vi "Restore Configuration.vi"(8 "error in (no error)":errorcluster, 10 "File path":path, 11 "Measure Object in":refnum<class "Template Module.lvclass">) -> (0 "error out":errorcluster, 1 "Section out":string, 2 "File path out":path, 3 "Measure Object out":refnum<class "Template Module.lvclass">)   [LabVIEW 2016, in "Template Module.lvclass"]
uses:
  Template Module.lvclass
  Template Module.lvclass/Template Module.ctl
  Read Name.vi
  Template Module Messages/Restore Configuration Msg/Restore Configuration Msg.lvclass
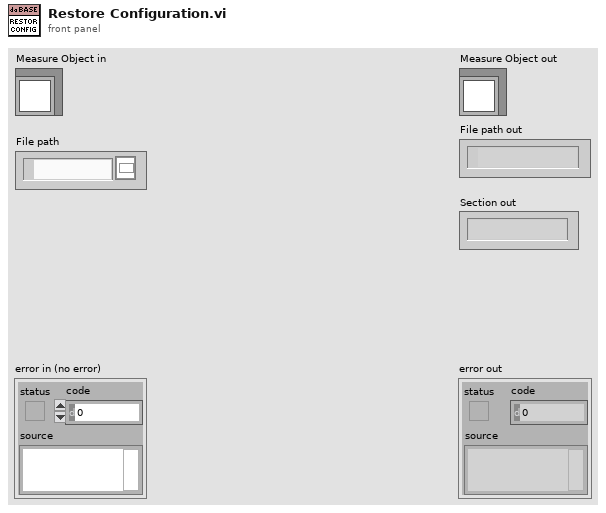
[diagram p1: front panel]
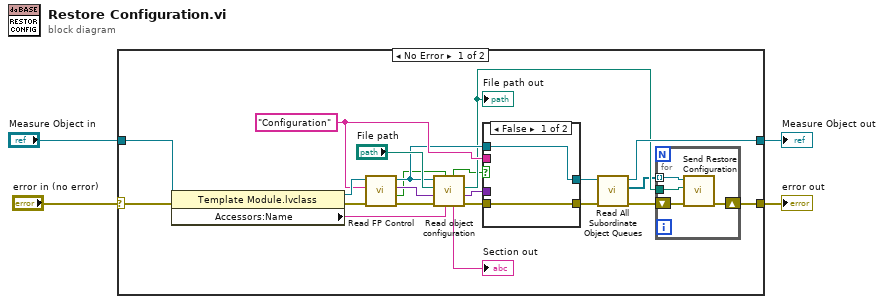
[diagram p0: block diagram]
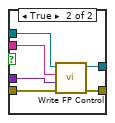
[diagram p2: hidden frame]
diagram:
  n1 = case shown="No Error" "error in (no error)" {
    selector: "error in (no error)" -> [w22 w40]
    tunnel: [w8 w40] -> w3
    tunnel: [w12 w39] -> w1
    tunnel: "Measure Object in" -> [w21 w39]
    frame No Error {
      w18 = "Configuration" ("Control Name")
      n2 = property class="Template Module.lvclass"(reference=w21, error in=w22) -> (reference out=w20:refnum<class "Template Module.lvclass">, error out=w23:errorcluster, "Accessors:Name"=w19:string)
      n3 = call-dynamic "Read FP Control.vi"("error in (no error)"=w23, "Control Name"=w18, "Measure Object in"=w20) -> ("error out"=w24:errorcluster, "Present"=w5:bool, "Control Value"=w26:variant, "Measure Object out"=w15:refnum<class "Template Module.lvclass">)  [unwired: 5 in]
      n4 = call "Read object configuration.vi"("Object name"=w19, "Present"=w5, "Error In"=w24, "type"=w26, "File path"="File path", "object"=w15) -> ("Error Out"=w16:errorcluster, "Configuration"=w17:variant, "File path out"=w11:path, "Section out"=→"Section out":string, "found?"=w6:bool)  [unwired: 1 in]
      "File path out" <- w11
      n5 = case shown="False" w6 {
        tunnel: w18 -> [_ w34]
        tunnel: w17 -> [_ w33]
        tunnel: w16 -> [w28 w32]
        tunnel: w15 -> [w27 w31]
        tunnel: [w28 w30] -> w14
        tunnel: [w27 w29] -> w13
        frame False {
        }
        frame True {
          n6 = call-dynamic "Write FP Control.vi"("error in (no error)"=w32, "Control Value"=w33, "Control Name"=w34, "Measure Object in"=w31) -> ("error out"=w30:errorcluster, "Measure Object out"=w29:refnum<class "Template Module.lvclass">)  [unwired: 6 in]
        }
      }
      n7 = call-dynamic "Read All Subordinate Object Queues.vi"("error in (no error)"=w14, "Measure Object in"=w13) -> ("error out"=w9:errorcluster, "Object enqueuers"=w10:refnum<class "Message Enqueuer.lvclass">[], "Measure Object out"=w12:refnum<class "Template Module.lvclass">)  [unwired: 6 in, 1 out]
      n8 = for {
        tunnel: w11 -> [w38]
        tunnel: w10 -> [w37] mode=indexing
        shift-right: [w36] -> w8
        shift-left: w9 -> [w35]
        n9 = call "Send Restore Configuration.vi"("error in (no error)"=w35, "File path"=w38, "Message Enqueuer"=w37) -> ("error out"=w36:errorcluster)  [unwired: 7 in, 1 out]
      }
    }
    frame Error {
    }
  }
  "error out" <- w3
  "Measure Object out" <- w1
